vi "Initialize.vi"(8 "error in (no error)":errorcluster, 9 "ID Query (T: Check)":bool=TRUE, 10 "Reset (T: Reset)":bool=TRUE, 11 "Tektronix PA1000 in":refnum<class "Tektronix PA1000.lvclass">) -> (0 "error out":errorcluster, 2 "VISA resource name":refnum<visa-resource-name>, 3 "Tektronix PA1000 out":refnum<class "Tektronix PA1000.lvclass">)   [LabVIEW 2016, in "Generic Power Analyzer.lvlib" / "Tektronix PA1000.lvlib" / "Tektronix PA1000.lvclass"]
uses:
  Tektronix PA1000.lvclass
  <instrlib>/Tektronix PA1000/Tektronix PA1000.lvlib
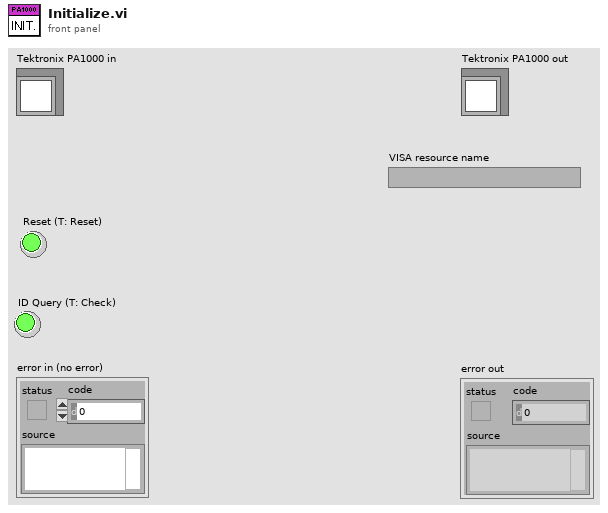
[diagram p1: front panel]
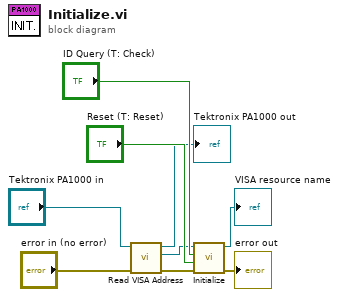
[diagram p0: block diagram]
diagram:
  n1 = call-dynamic "Read VISA Address.vi"("error in (no error)"="error in (no error)", "Generic Device in"="Tektronix PA1000 in") -> ("error out"=w1:errorcluster, "VISA Address"=w3:refnum<visa-resource-name>, "Generic Device out"=→"Tektronix PA1000 out":refnum<class "Tektronix PA1000.lvclass">)  [unwired: 7 in]
  n2 = call <instrlib>:"Initialize.vi"("error in (no error)"=w1, "Reset (True)"="Reset (T: Reset)", "ID Query (True)"="ID Query (T: Check)", "VISA resource name"=w3) -> ("error out"=→"error out":errorcluster, "VISA resource name out"=→"VISA resource name":refnum<visa-resource-name>)  [unwired: 6 in]
